vi "Abs.vi"(8 "error in":errorcluster, 11 "Vec3d in":refnum<class "Vec3d.lvclass">) -> (0 "error out":errorcluster, 3 "Vec3d out":refnum<class "Vec3d.lvclass">)   [LabVIEW 2022 SP3, in "Vec3d.lvclass"]
uses:
  Vec3d.lvclass
  Vec3d.lvclass/Vec3d.ctl
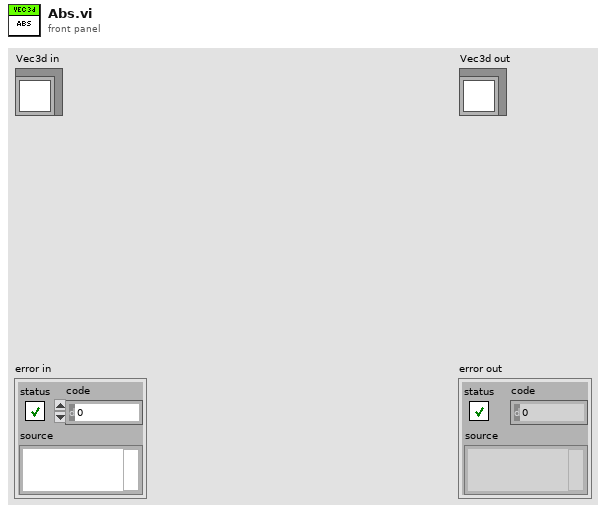
[diagram p1: front panel]
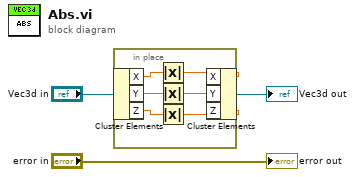
[diagram p0: block diagram]
diagram:
  n1 = in-place {
    n2 = in-place-cluster #1("Vec3d in") -> ("X"=w8:dbl, "Y"=w9:dbl, "Z"=w7:dbl)
    n3 = Absolute Value(x=w8) -> (abs(x)=w6:dbl)
    n4 = Absolute Value(x=w9) -> (abs(x)=w5:dbl)
    n5 = Absolute Value(x=w7) -> (abs(x)=w4:dbl)
    n6 = in-place-cluster #1("X"=w6, "Y"=w5, "Z"=w4) -> (→"Vec3d out":refnum<class "Vec3d.lvclass">)
  }
  "error out" <- "error in"
